vi "getInputGain.vi"(8 "error in (no error)":errorcluster, 11 "Instrument.LockinAPI in":refnum<class "Instrument.LockinAPI.lvclass">) -> (0 "error out":errorcluster, 2 "InputGain":dbl[](array[numeric]), 3 "Instrument.LockinAPI out":refnum<class "Instrument.LockinAPI.lvclass">)   [LabVIEW 2019, in "Instrument.LockinAPI.lvclass"]
doc: "API to get the gain at the input\n\nIf address=\"\", this API reads from localhost\nIf address is remote lockin, you need to add this computer to allowed whitelist on the lockin computer you are trying to access."
uses:
  Instrument.LockinAPI.lvclass
  C:/Users/patrick/Documents/GitHub/Instrument-Framework/lvsrc/Framework/Instrument/Instrument.lvclass
  Typedefs/LockinAPI.commands--Enum.ctl
  4cd01352-97e2-4cf3-bc9b-89122dc6c5e8.vi
  4cd01352-97e2-4cf3-bc9b-89122dc6c5e8.vi/97eeb512-01e2-4811-978c-0ce28ae61649.vi
  4cd01352-97e2-4cf3-bc9b-89122dc6c5e8.vi/b58e276f-8985-45b0-aeaf-0f97e475fd12.vi
  <vilib>/Utility/Data Type/Get Type Information.vi
  <vilib>/JDP Science/JSONtext/JSON text to Variant.vi
  <vilib>/JDP Science/JSONtext/LVClass Serializer/JSONtext LVClass Serializer.lvclass
  Instrument/Instrument.lvclass
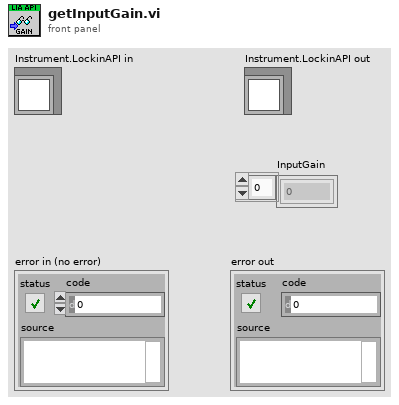
[diagram p1: front panel]
types:
  T1 = typedef "Instrument.LockinAPI.lvclass/LockinAPI.commands--Enum.ctl" = enum16{"setAI", "setAO", "setAO_Amplitude", "setAO_DC", "setAO_Frequency", "setAO_Phase", "setAO_Function", "setAO_I+", "setREF", "setREF_Frequency", "setREF_Phase", "setREF_TC", "setREF_Roll-Off", "setDAQ", "setSampling", "setOffset", "setState", "getState", "getAO", "getAI", "getResults", "getSampling", "getAOconfig", "getREFconfig", "setInputGain", "setOutputGain", "getInputGain", "getOutputGain", "setSamplingMode", "getSamplingMode", "setSweep", "setSweepTime", "setSweepTable", "getStatus", "getSweepResults", "getSweepWaveforms", "startSweep", "stopSweep", "setAUX", "getAUX"}
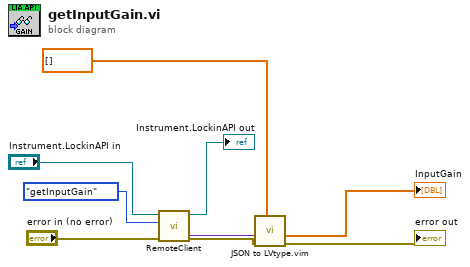
[diagram p0: block diagram]
diagram:
  n1 = call "RemoteClient.vi"("error in (no error)"="error in (no error)", "Command in"=LockinAPI.commands--Enum."getInputGain" ("Command"), "Instrument in"="Instrument.LockinAPI in") -> ("error out"=w4:errorcluster, "Data out"=w3:variant, "Instrument out"=→"Instrument.LockinAPI out":refnum<class "Instrument.LockinAPI.lvclass">)  [unwired: 5 in, 1 out]
  n2 = call "JSON to LVtype.vim"("type"=dbl[] [] ("InputGain"), "error in (no error)"=w4, "JSON Data in"=w3) -> ("error out"=→"error out":errorcluster, "Data out"=→"InputGain":dbl[])  [unwired: 7 in]
